vi "Test Get All.vi"(6 "Descending? (F)":bool, 8 "error in (no error)":errorcluster, 10 "Sort by (sxTestId)":T1, 11 "Connection Refnum":T2) -> (0 "error out":errorcluster, 2 "Test Records":T3[](array[typedef]), 3 "Connection Refnum":T2, 4 "Data Present":bool)   [LabVIEW 2011]
uses:
  Test Record.ctl
  Summitek EXT/ODBC/SQL Controls/Connection Refnum.ctl
  Test Table Fields.ctl
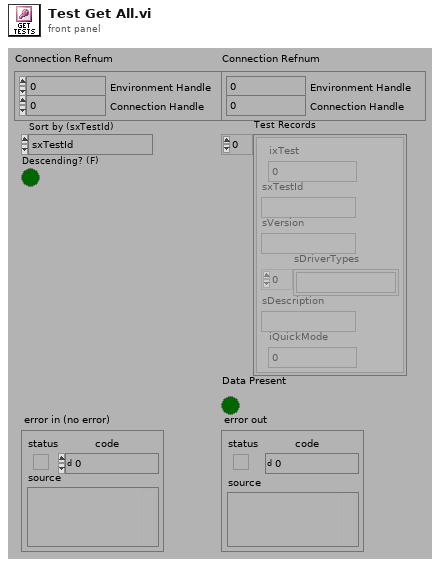
[diagram p1: front panel]
types:
  T1 = typedef "Test Table Fields.ctl" = enum32{"sxTestId", "sVersion", "sDriverTypes", "sDescription", "sQuickMode", "ixTest"}
  T2 = typedef "Connection Refnum.ctl" = cluster{"Environment Handle":i32, "Connection Handle":i32}
  T3 = typedef "Test Record.ctl" = cluster{"ixTest":i32, "sxTestId":string, "sVersion":string, "sDriverTypes":string[], "sDescription":string, "iQuickMode":i32}
  T4 = typedef "Statement Refnum.ctl" = cluster{"Statement Handle":i32, "Parameter Number":u16}
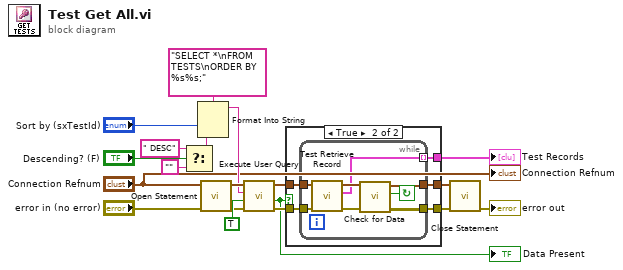
[diagram p0: block diagram]
diagram:
  n1 = Select(t=" DESC" ("input 2"), s="Descending? (F)", f="") -> (s? t:f=w9:string)
  n2 = Format Into String(format string="SELECT *\nFROM TESTS\nORDER BY %s%s;" ("Query Name"), "Sort by (sxTestId)", w9) -> (resulting string=w5:string)  [unwired: 2 in, 1 out]
  n3 = call "Open Statement.vi"("error in (no error)"="error in (no error)", "Connection Refnum"="Connection Refnum") -> ("error out"=w13:errorcluster, "Statement Refnum"=w14:T4)  [unwired: 4 out]
  n4 = call "Execute User Query.vi"("error in (no error)"=w13, "Return Data? (f)"=TRUE, "User Query"=w5, "Statement Refnum"=w14) -> ("error out"=w19:errorcluster, "Data Present?"=w12:bool, "Statement Refnum"=w18:T4)  [unwired: 1 out]
  "Data Present" <- w12
  n5 = case shown="True" w12 {
    tunnel: w19 -> [w20 w25]
    tunnel: w18 -> [w21 w26]
    tunnel: [w20 w23] -> w15
    tunnel: [w21 w24] -> w16
    tunnel: [_ w22] -> w3
    frame False {
    }
    frame True {
      n6 = while {
        tunnel: w26 -> [w33]
        tunnel: w25 -> [w32]
        tunnel: [w30] -> w24
        tunnel: [w28] -> w23
        tunnel: [w27] -> w22 mode=indexing
        stop <- w34 continue-if-true
        n7 = call "Test Retrieve Record.vi"("error in (no error)"=w32, "Statement Refnum"=w33) -> ("error out"=w29:errorcluster, "Test Record"=w27:T3, "Statement Refnum"=w31:T4)  [unwired: 7 out]
        n8 = call "Check for Data.vi"("error in (no error)"=w29, "Statement Refnum"=w31) -> ("error out"=w28:errorcluster, "Data Present?"=w34:bool, "Statement Refnum"=w30:T4)  [unwired: 3 out]
      }
    }
  }
  "Test Records" <- w3
  n9 = call "Close Statement.vi"("error in (no error)"=w15, "Statement Refnum"=w16) -> ("error out"=→"error out":errorcluster)  [unwired: 5 out]
  "Connection Refnum" <- "Connection Refnum"
